vi "VISA WRITE&READ.vi"(5 "byte count":u32, 7 "Delay(mS)":u32, 8 "error in (no error)":errorcluster, 9 "Read?":bool, 10 "write buffer":string, 11 "VISA resource name In":refnum<visa-resource-name>) -> (0 "error out":errorcluster, 2 "read buffer":string, 3 "VISA resource name Out":refnum<visa-resource-name>)   [LabVIEW 2018]
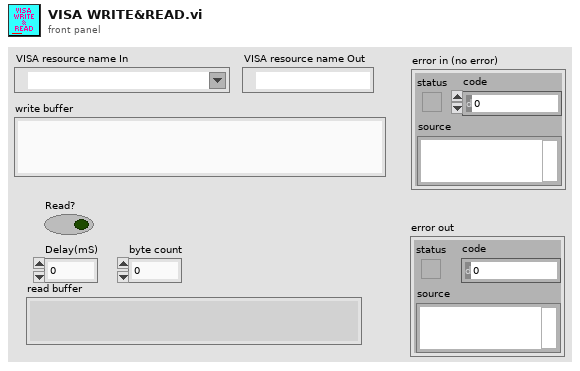
[diagram p1: front panel]
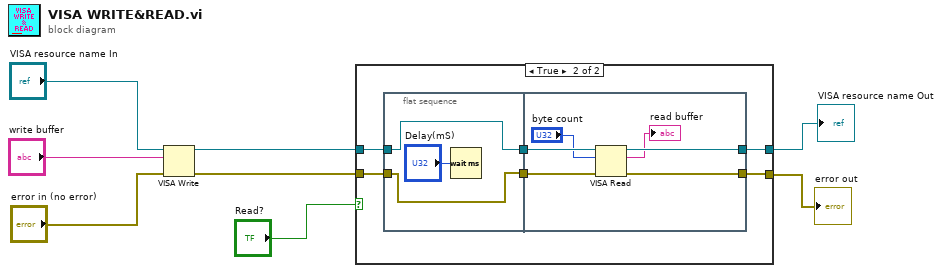
[diagram p0: block diagram]
diagram:
  n1 = VISA Write(VISA resource name="VISA resource name In", write buffer="write buffer", error in (no error)="error in (no error)") -> (VISA resource name out=w4:refnum<visa-resource-name>, error out=w3:errorcluster)  [unwired: 1 out]
  n2 = case shown="True" "Read?" {
    tunnel: w4 -> [w10 w16]
    tunnel: w3 -> [w9 w14]
    tunnel: [w10 w12] -> w1
    tunnel: [w9 w11] -> w2
    frame False {
    }
    frame True {
      n3 = flat-sequence {
        tunnel: w16 -> [w18]
        tunnel: [w18] -> w15
        tunnel: w14 -> [w17]
        tunnel: [w17] -> w13
        tunnel: w15 -> [w25]
        tunnel: w13 -> [w24]
        tunnel: [w22] -> w12
        tunnel: [w20] -> w11
        frame #0 {
          n4 = Wait (ms)(milliseconds to wait="Delay(mS)") -> ()  [unwired: 1 out]
        }
        frame #1 {
          n5 = VISA Read(VISA resource name=w25, byte count="byte count", error in (no error)=w24) -> (VISA resource name out=w22:refnum<visa-resource-name>, read buffer=→"read buffer":string, error out=w20:errorcluster)  [unwired: 1 out]
        }
      }
    }
  }
  "error out" <- w2
  "VISA resource name Out" <- w1
